vi "Untitled 15.vi"() -> ()   [LabVIEW 2017]
uses:
  <vilib>/Utility/Data Type/Type Definitions/Data Type.ctl
  <vilib>/Utility/Data Type/Type Definitions/Refnum Type.ctl
  cf12a62b-1720-4f19-8a00-076dd31e3abf.vi
  3c156090-785c-496c-b4e3-754212adb3b2.vi
  addons/API-String-Arugments-Support/_Support/Query Data as API String Arguments(variant).vi
  <vilib>/Utility/Data Type/NI_Data Type.lvlib
  <userlib>/_NEVSTOP/Communicable State Machine(CSM)/_Shared/CSM Shared.lvlib
  addons/API-String-Arugments-Support/API String Arguments Support.lvlib
panel:
  in  "output cluster":T1={"Core"={"Current VI Reference"=refnum, "Close Panel on Exit?"=FALSE, "Settings"=FALSE}, "DataBool"=FALSE, "DataString"="asdfa", "cluster"={"Bool"=FALSE, "string"="asdfasf", "Settings"={"Bool"=FALSE, "string"="asdfasdf", "Settings"="asdfasdf"}, "Settings 2"=FALSE}}
  out "<list>":string
  out "API String":string
  in  "Name":string
  out "Array 2":i32[](array[numeric])
  out "Array":string[](array[string])
  out "DataElementArray":variant[](array[variant])
  out "Type 3":T2
  out "Reference Type 2":T3
  out "Type 2":T2
  out "Reference Type":T3
  out "Type":T2
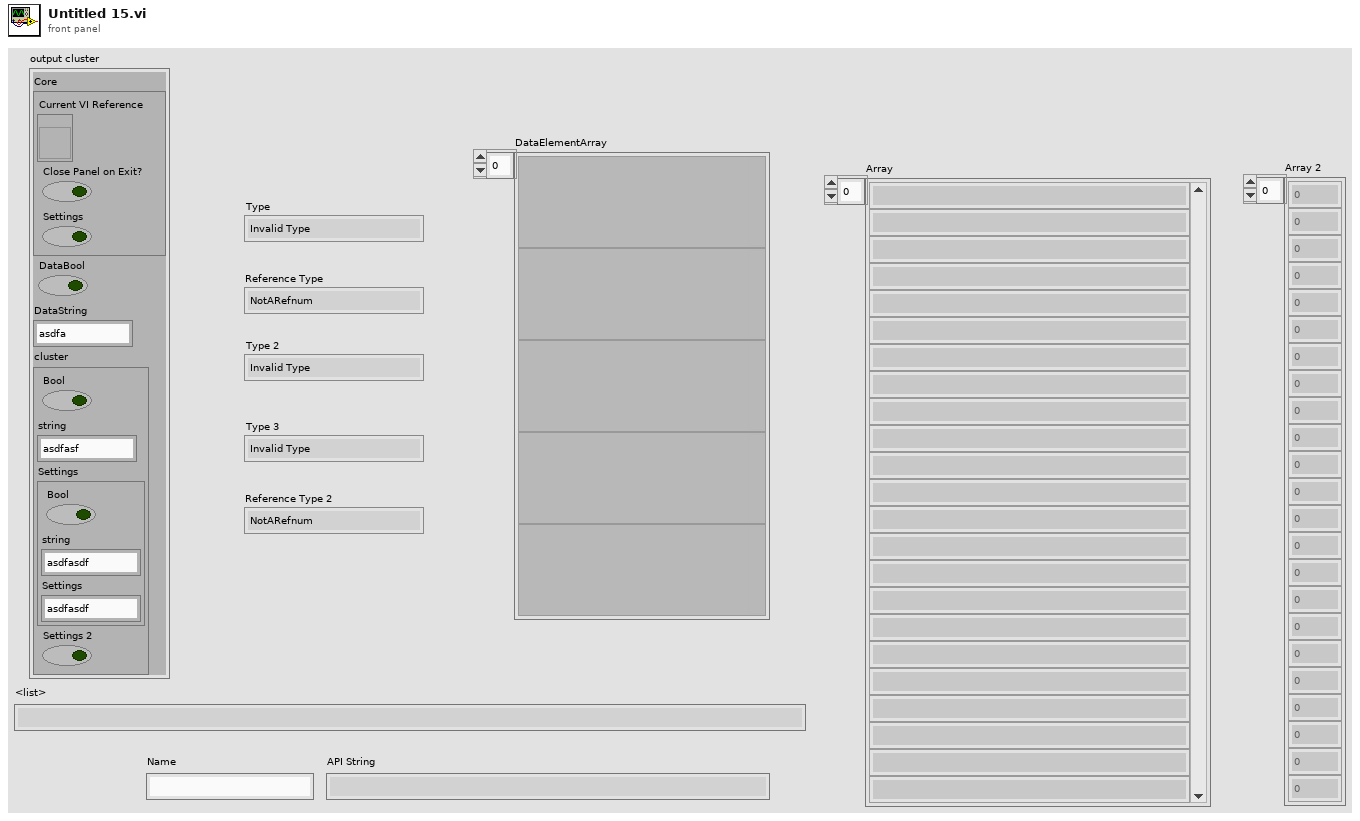
[diagram p1: front panel]
types:
  T1 = cluster{"Core":cluster{"Current VI Reference":refnum<vi>, "Close Panel on Exit?":bool, "Settings":bool}, "DataBool":bool, "DataString":string, "cluster":cluster{"Bool":bool, "string":string, "Settings":cluster{"Bool":bool, "string":string, "Settings":string}, "Settings 2":bool}}
  T2 = typedef "NI_Data Type.lvlib/Data Type.ctl" = enum8{"Invalid Type", "Void", "I8", "I16", "I32", "I64", "U8", "U16", "U32", "U64", "Single Float", "Double Float", "Extended Float", "Single Complex", "Double Complex", "Extended Complex", "Enum U8", "Enum U16", "Enum U32", "Enum U64", "Single Float With Unit", "Double Float With Unit", "Extended Float With Unit", "Single Complex with Unit", "Double Complex with Unit", "Extended Complex with Unit", "Boolean", "String", "Path", "Picture", "Tag", "Array", "Cluster", "Variant", "LV Variant", "Waveform", "Timestamp", "Digital Waveform", "Digital Data", "ExpressData", "Refnum", "External Data", "VI", "Poly VI", "LabVIEW Class Instance", "Fixed Point"}
  T3 = typedef "NI_Data Type.lvlib/Refnum Type.ctl" = enum16{"NotARefnum", "UnknownRefnum", "Generic", "Datalog", "ByteStream", "Device", "Occurence", "TCPNetConnection", "Auto", "Menu", "Imaq", "Hardware", "DataSocket", "Visa", "IVI", "UDPNetConnection", "Notifier", "Queue", "Irda", "EventReg", "DotNet", "UserEvent", "Callback", "UNUSED_EMPTY_POSITION", "BlueToothNetConnection", "LVObjApp", "LVObjVI", "LVObjUnknown", "GenericClass", "UserDefinedRefnumTag", "DataValue", "RT FIFO", "TDMS File"}
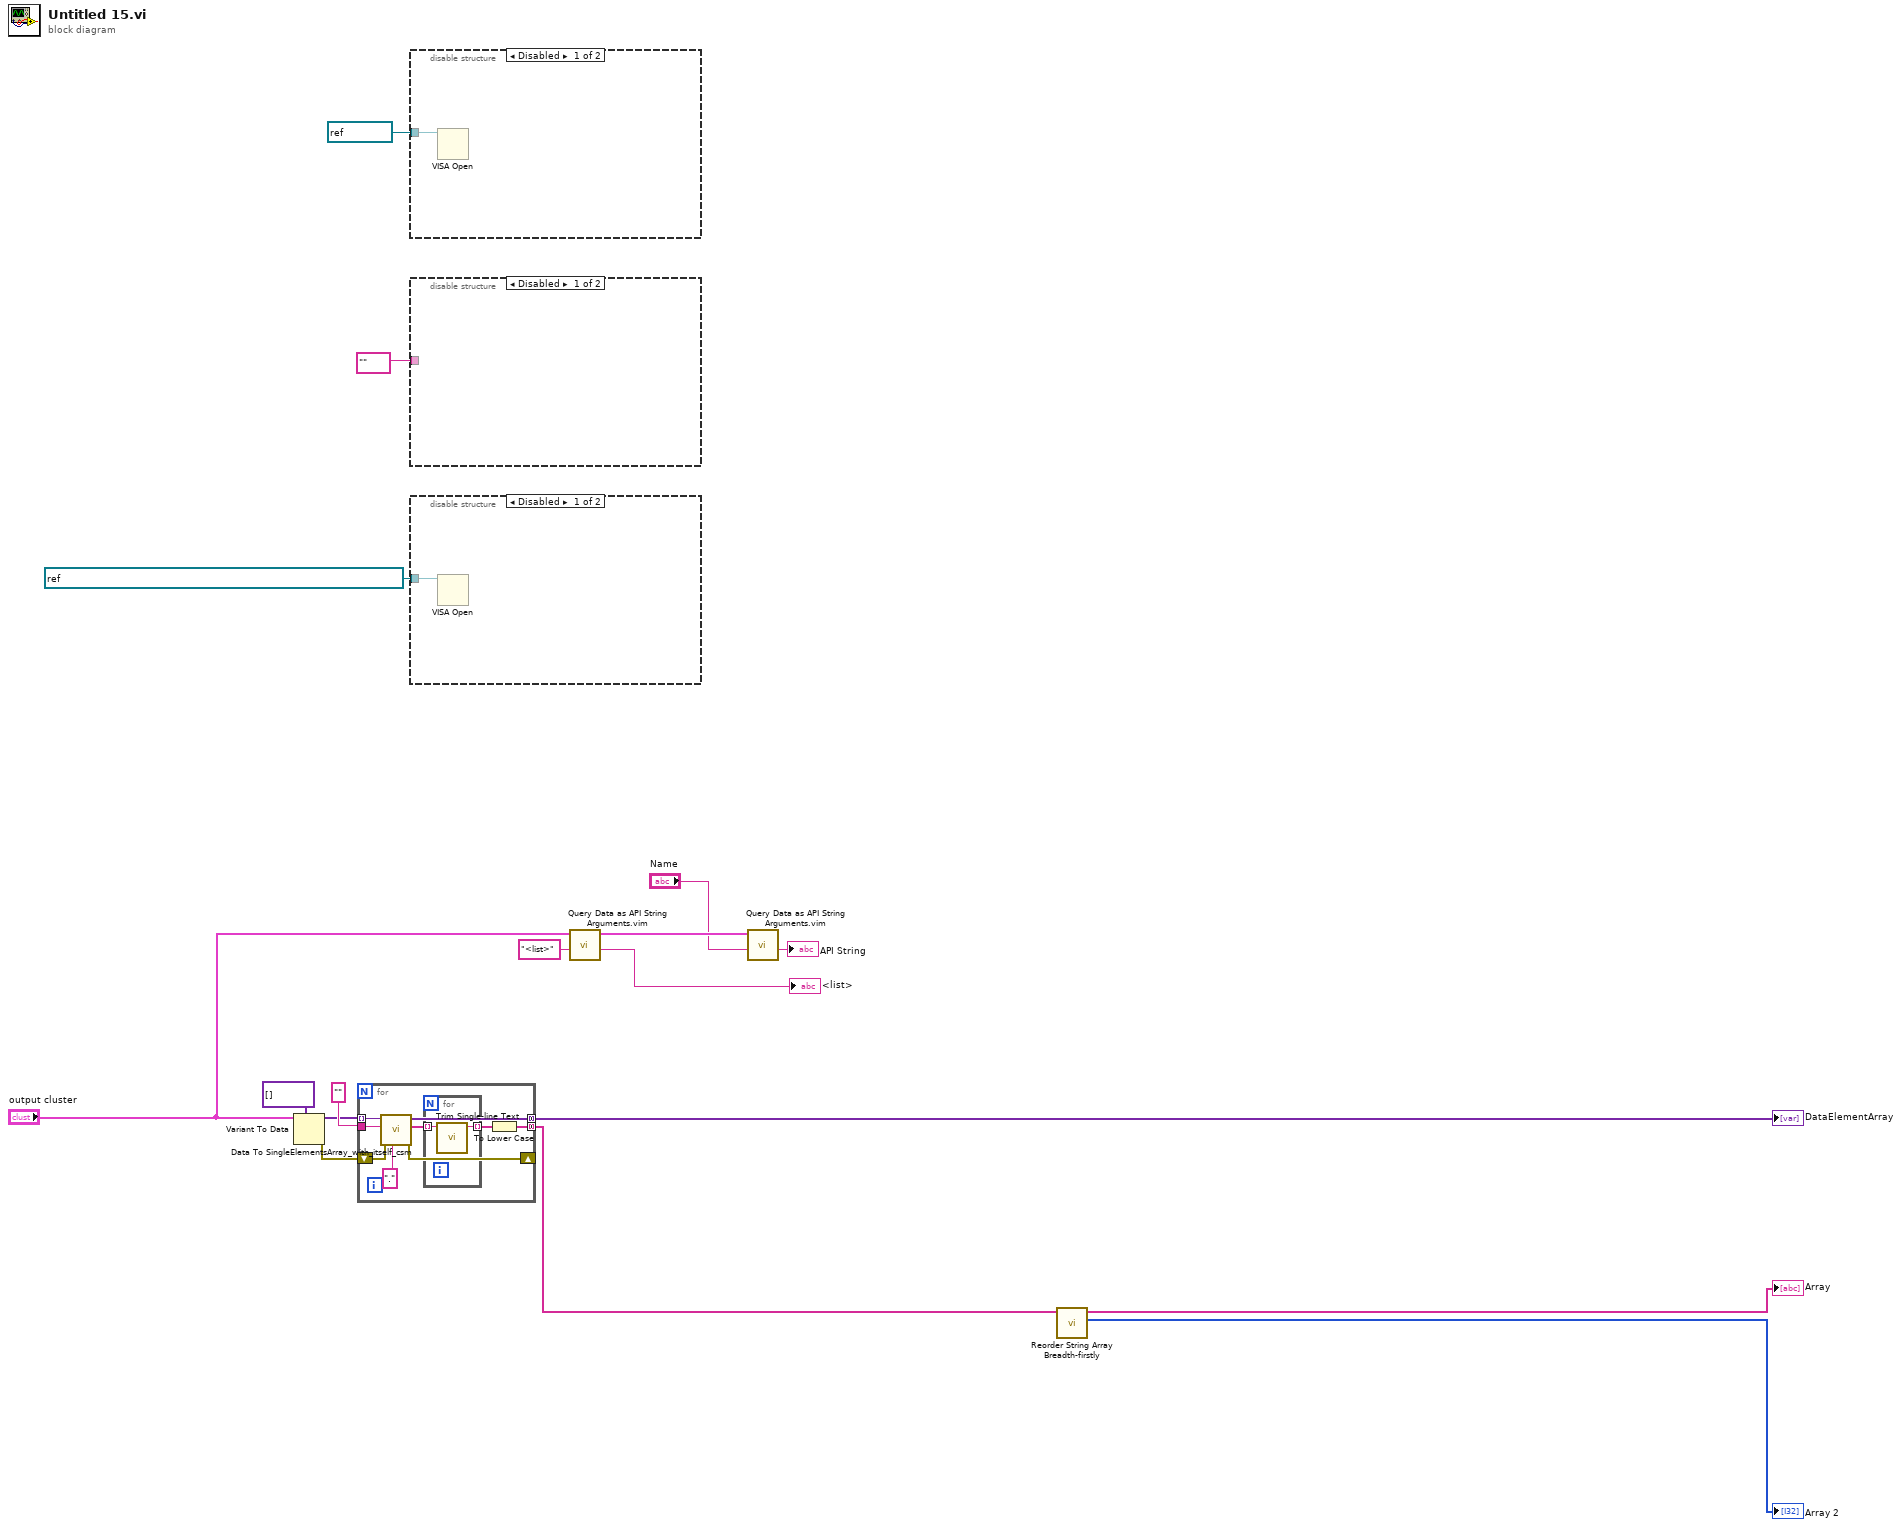
[diagram p0: block diagram]
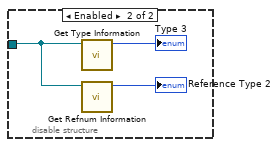
[diagram p2: hidden frame]
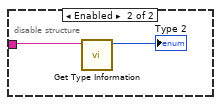
[diagram p3: hidden frame]
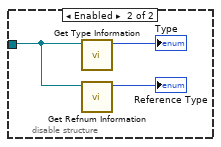
[diagram p4: hidden frame]
diagram:
  n1 = Variant To Data(type=variant[] [] ("Array"), Variant="output cluster") -> (data=w12:variant[], error out=w11:errorcluster)  [unwired: 1 in]
  n2 = for {
    tunnel: [w24] -> w10 mode=concatenating
    tunnel: [w18] -> w9 mode=concatenating
    tunnel: "" ("parentUrl") -> [w21]
    tunnel: w12 -> [w20] mode=indexing
    shift-right: [w23] -> _
    shift-left: w11 -> [w26]
    n3 = call "Data To SingleElementsArray_with_itself_csm.vi"("Seperator(/)"=".", "error in (no error)"=w26, "parentUrl"=w21, "Cluster"=w20) -> ("error out"=w23:errorcluster, "Full NameList"=w22:string[], "DataElementArray"=w24:variant[])  [unwired: 5 in]
    n4 = for {
      tunnel: w22 -> [w28] mode=indexing
      tunnel: [w27] -> w19 mode=indexing
      n5 = call <userlib>:"Trim Single-line Text.vi"("single-line text"=w28) -> ("trimed text"=w27:string)  [unwired: 2 in]
    }
    n6 = To Lower Case(string=w19) -> (all lower case string=w18:string[])
  }
  "DataElementArray" <- w10
  n7 = disable-structure shown="Disabled" {
    disable-tunnel: refnum<visa-resource-name> "COM3" ("VISA resource name") -> [w29 w31]
    frame Disabled {
      n8 = VISA Open(VISA resource name=w29) -> ()  [unwired: 4 in, 2 out]
    }
    frame Enabled {
      n9 = call <vilib>:"Get Type Information.vi"("Variant"=w31) -> ("Type"=→"Type":T2)  [unwired: 6 in, 4 out]
      n10 = call <vilib>:"Get Refnum Information.vi"("Variant"=w31) -> ("Reference Type"=→"Reference Type":T3)  [unwired: 7 in, 3 out]
    }
  }
  n11 = disable-structure shown="Disabled" {
    disable-tunnel: tag "" ("Device Name") -> [_ w33]
    frame Disabled {
    }
    frame Enabled {
      n12 = call <vilib>:"Get Type Information.vi"("Variant"=w33) -> ("Type"=→"Type 2":T2)  [unwired: 6 in, 4 out]
    }
  }
  n13 = disable-structure shown="Disabled" {
    disable-tunnel: refnum<k21> "ni.var.psp://localhost/System/DAQmx/Server Polling Rate" ("shared variable refnum in") -> [w35 w37]
    frame Disabled {
      n14 = VISA Open(VISA resource name=w35) -> ()  [unwired: 4 in, 2 out]
    }
    frame Enabled {
      n15 = call <vilib>:"Get Type Information.vi"("Variant"=w37) -> ("Type"=→"Type 3":T2)  [unwired: 6 in, 4 out]
      n16 = call <vilib>:"Get Refnum Information.vi"("Variant"=w37) -> ("Reference Type"=→"Reference Type 2":T3)  [unwired: 7 in, 3 out]
    }
  }
  n17 = call "Query Data as API String Arguments.vim"("Name"="<list>", "Cluster Data"="output cluster") -> ("API String"=→"<list>":string, "Cluster Data (dup)"=w4:T1)  [unwired: 7 in, 1 out]
  n18 = call "Query Data as API String Arguments.vim"("Name"="Name", "Cluster Data"=w4) -> ("API String"=→"API String":string)  [unwired: 7 in, 2 out]
  n19 = call "Reorder String Array Breadth-firstly.vi"("Array 3"=w9) -> ("Indexs"=→"Array 2":i32[], "Array"=→"Array":string[])  [unwired: 9 in]
